vi "Fetch Waveforms.vi"(8 "error in":errorcluster, 11 "Fetch Display CFG in":refnum<class "Fetch Display CFG.lvclass">) -> (0 "error out":errorcluster, 2 "Last Waveforms":map{u8, waveform(dbl)}(c390), 3 "Fetch Display CFG out":refnum<class "Fetch Display CFG.lvclass">)   [LabVIEW 2023, in "Fetch Display CFG.lvclass"]
uses:
  Fetch Display CFG.lvclass
  Fetch Display CFG.lvclass/Fetch Display CFG.ctl
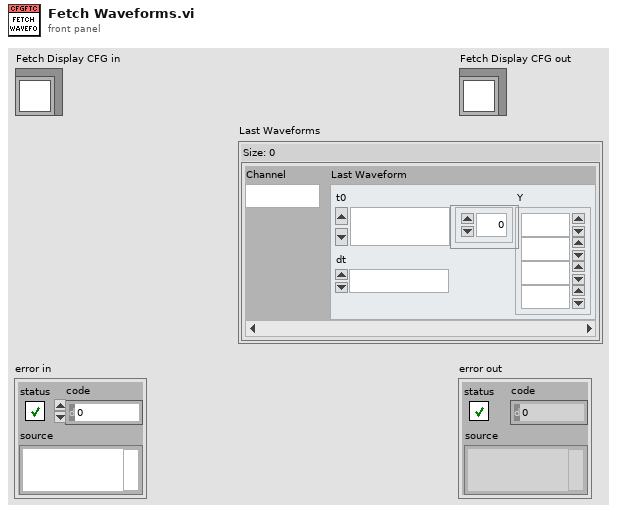
[diagram p1: front panel]
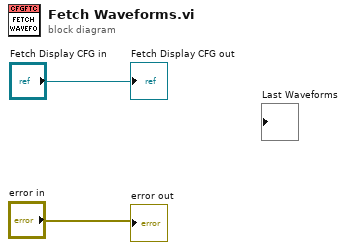
[diagram p0: block diagram]
diagram:
  "error out" <- "error in"
  "Fetch Display CFG out" <- "Fetch Display CFG in"
